vi "Eingabe Nominal Point.vi"() -> (2 "NominaPoint":T1={"Punktnummer"="", "Transformation Point"={"dVal1"=0.0, "dVal2"=0.0, "dVal3"=0.0, "dStd1"=0.0001, "dStd2"=0.0001, "dStd3"=0.0001, "dCovar12"=0.0, "dCovar13"=0.0, "dCovar23"=0.0}})   [LabVIEW 2017]
uses:
  AT901 API/Structures/Struct TransformationPointWithPointnumber.ctl
  AT901 API/Structures/Struct TransformationPoint.ctl
panel:
  in  "Punktnummer":string
  in  "stop":bool
  in  "Z - Koordinate":dbl
  in  "Y - Koordinate":dbl
  in  "X - Koordinate":dbl
  # "Bitte Koordinate \n(nominal Point) eingeben!"
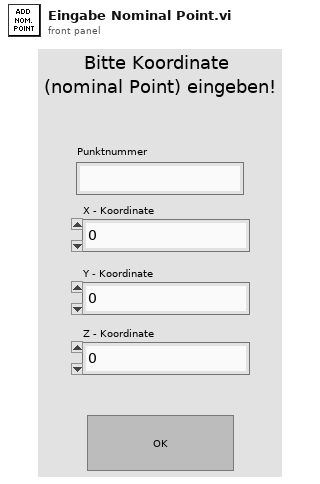
[diagram p1: front panel]
types:
  T1 = typedef "Struct TransformationPointWithPointnumber.ctl" = cluster{"Punktnummer":string, "Transformation Point":T2}
  T2 = typedef "Struct TransformationPoint.ctl" = cluster{"dVal1":dbl, "dVal2":dbl, "dVal3":dbl, "dStd1":dbl, "dStd2":dbl, "dStd3":dbl, "dCovar12":dbl, "dCovar13":dbl, "dCovar23":dbl}
  T3 = cluster{"Punktnummer":string, "Transformation Point":T2}
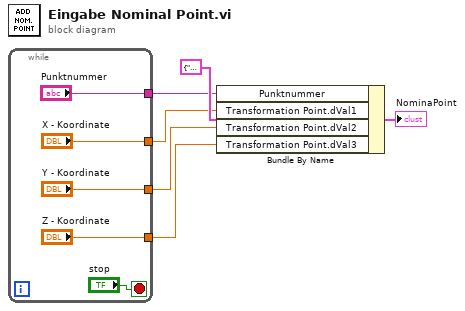
[diagram p0: block diagram]
diagram:
  n1 = while {
    tunnel: ["Punktnummer"] -> w4
    tunnel: ["X - Koordinate"] -> w3
    tunnel: ["Y - Koordinate"] -> w2
    tunnel: ["Z - Koordinate"] -> w1
    stop <- "stop" stop-if-true
  }
  n2 = Bundle By Name(cluster=T3 {"Punktnummer"="", "Transformation Point"={"dVal1"=0.0, "dVal2"=0.0, "dVal3"=0.0, "dStd1"=0.0, "dStd2"=0.0, "dStd3"=0.0, "dCovar12"=0.0, "dCovar13"=0.0, "dCovar23"=0.0}} ("Actual Point"), "Punktnummer"=w4, "Transformation Point.dVal1"=w3, "Transformation Point.dVal2"=w2, "Transformation Point.dVal3"=w1) -> (→"NominaPoint":T3)
